vi "Exercise_3-5_Liam_Hubbard.vi"() -> ()   [LabVIEW 2014]
panel:
  in  "Current Temp":dbl
  in  "Max Temp":dbl
  in  "Min Temp":dbl
  out "Warning Text":string
  out "Warning?":bool
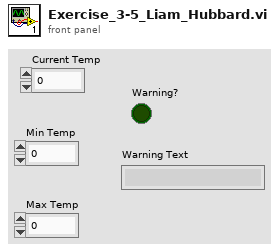
[diagram p1: front panel]
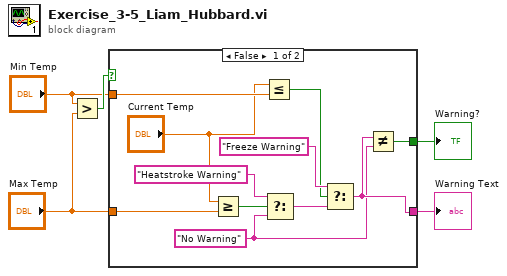
[diagram p0: block diagram]
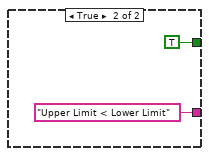
[diagram p2: hidden frame]
diagram:
  n1 = Greater?(x="Min Temp", y="Max Temp") -> (0:w5:bool)
  n2 = case shown="False" w5 {
    tunnel: "Min Temp" -> [w7 _]
    tunnel: "Max Temp" -> [w16 _]
    tunnel: [w15 "Upper Limit < Lower Limit"] -> w2
    tunnel: [w8 TRUE] -> w1
    frame False {
      w11 = "No Warning"
      n3 = Greater Or Equal?(x="Current Temp", y=w16) -> (x >= y?=w10:bool)
      n4 = Less Or Equal?(x="Current Temp", y=w7) -> (x <= y?=w12:bool)
      n5 = Select(t="Heatstroke Warning", s=w10, f=w11) -> (s? t:f=w13:string)
      n6 = Select(t="Freeze Warning", s=w12, f=w13) -> (s? t:f=w15:string)
      n7 = Not Equal?(x=w15, y=w11) -> (x != y?=w8:bool)
    }
    frame True {
    }
  }
  "Warning Text" <- w2
  "Warning?" <- w1
